vi "night.vi"() -> ()   [LabVIEW 2020]
uses:
  <vilib>/Analysis/baseanly.llb/Mean (DBL).vi
  <vilib>/Analysis/NI_AALBase.lvlib
panel:
  out "Error Out":errorcluster
  in  "milliseconds to wait":u32
  out "XY Graph":cluster{timestamp[], dbl[]}[](graph)
  in  "stop":bool
  out "Output":T1={"X"=[-0.192], "Y"=[-0.056], "Z"=[0.117], "Temperature"=0, "Timestamp"=525.141756172, "Digits"=3} {"Z" format="%.5f"; "Y" format="%.5f"; "X" format="%.5f"}
  in  "Select":T2={"X"=TRUE, "Y"=TRUE, "Z"=TRUE, "Temp"=FALSE, "Timstamp"=FALSE}
  out "File Error Out":errorcluster
  in  "COMMENT":string="BDC_z_reverse_D1_0A_D2_0A_SFDC_3A5"
  in  "base path":path=path "C:/LabVIEW/DATA/J-PARC_202403"
  in  "VISA resource":refnum<visa-resource-name>="USB0::0x1BFA::0x0498::0002759::INSTR"
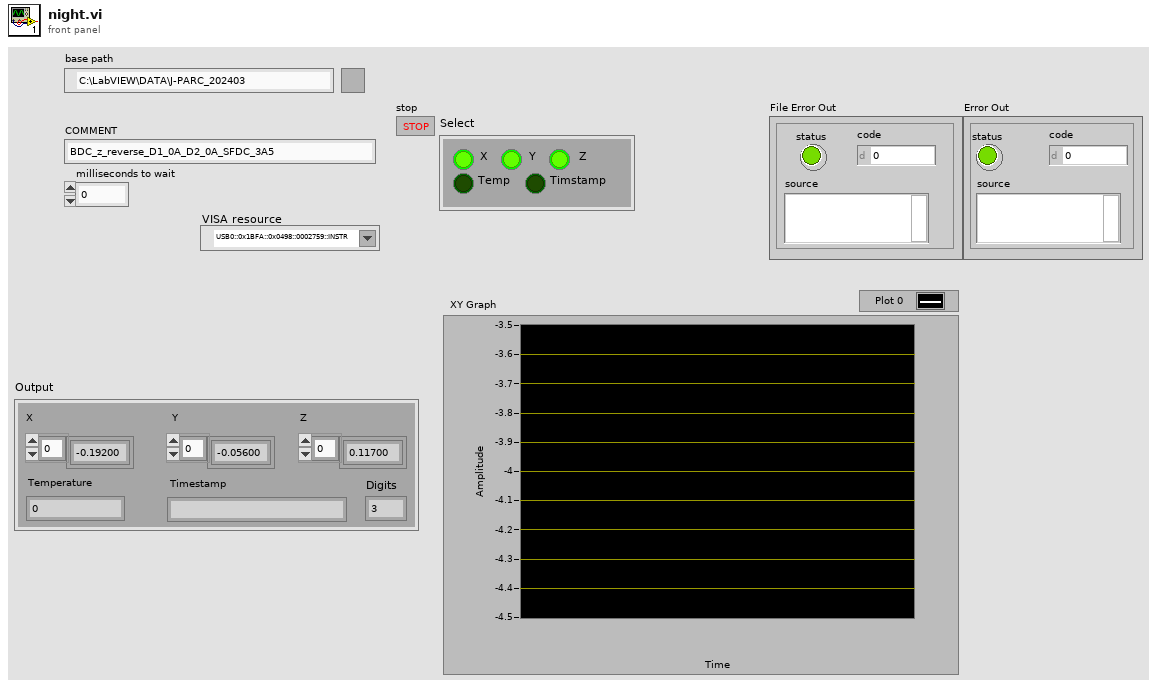
[diagram p1: front panel]
types:
  T1 = cluster{"X":dbl[], "Y":dbl[], "Z":dbl[], "Temperature":u16, "Timestamp":ext, "Digits":u8}
  T2 = cluster{"X":bool, "Y":bool, "Z":bool, "Temp":bool, "Timstamp":bool}
  T3 = enum16{"open", "replace", "create", "open or create", "replace or create", "replace or create with confirmation"}
  T4 = enum16{"Setup", "Setup query", "INITiate", "ABORt"}
  T5 = enum16{"Set units", "Units query", "Units all query"}
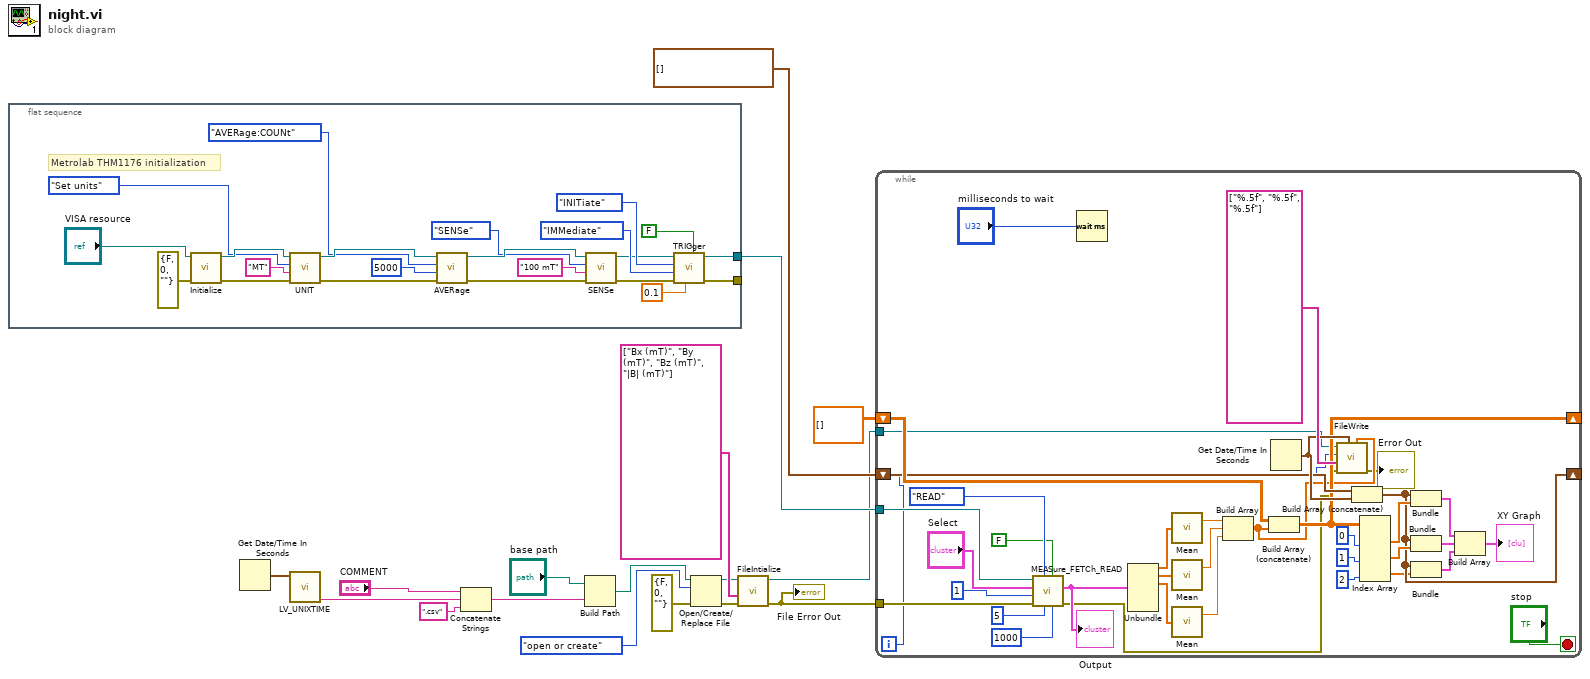
[diagram p0: block diagram]
diagram:
  n1 = flat-sequence {
    tunnel: [w25] -> w5
    tunnel: [w24] -> _
    frame #0 {
      # "Metrolab THM1176 initialization"
      n2 = call "Initialize.vi"("Error in (no error)"=errorcluster {"status"=FALSE, "code"=0, "source"=""}, "VISA resource"="VISA resource") -> ("Error out"=w36:errorcluster, "Dup VISA resource"=w37:refnum<visa-resource-name>)  [unwired: 3 in, 5 out]
      n3 = call "UNIT.vi"("Error in (no error)"=w36, "Units"="MT", "Function"=T5."Set units", "VISA resource"=w37) -> ("Error out"=w32:errorcluster, "Dup VISA resource"=w33:refnum<visa-resource-name>)  [unwired: 5 in, 1 out]
      n4 = call "AVERage.vi"("Error in (no error)"=w32, "Count"=u16 5000, "Function"=enum16{"AVERage:COUNt query", "AVERage:COUNt"}."AVERage:COUNt", "VISA resource"=w33) -> ("Error out"=w23:errorcluster, "Dup VISA resource"=w20:refnum<visa-resource-name>)  [unwired: 5 in, 1 out]
      n5 = call "SENSe.vi"("Error in (no error)"=w23, "Range"="100 mT", "Function"=enum16{"SENSe", "SENSe Query"}."SENSe", "VISA resource"=w20) -> ("Error out"=w22:errorcluster, "Dup VISA resource"=w21:refnum<visa-resource-name>)  [unwired: 4 in, 2 out]
      n6 = call "TRIGger.vi"("Continuous"=FALSE, "Period (s)"=0.1, "Error in (no error)"=w22, "Source"=enum16{"IMMediate", "TIMer", "BUS"}."IMMediate", "Function"=T4."INITiate", "VISA resource"=w21) -> ("Error out"=w24:errorcluster, "Dup VISA resource"=w25:refnum<visa-resource-name>)  [unwired: 3 in, 1 out]
    }
  }
  n7 = Get Date/Time In Seconds() -> (seconds since 1Jan1904=w15:timestamp)
  n8 = call "LV_UNIXTIME.vi"("current time"=w15) -> ("date/time string"=w12:string)  [unwired: 9 in, 1 out]
  n9 = Concatenate Strings("COMMENT", w12, ".csv" ("string")) -> (w10:string)
  n10 = Build Path(base path="base path", name or relative path=w10) -> (appended path=w14:path)
  n11 = Open/Create/Replace File(file path (use dialog)=w14, error in=errorcluster {"status"=FALSE, "code"=0, "source"=""} ("エラー入力"), operation (0:open)=T3."open or create") -> (refnum out=w7:refnum<file>, error out=w8:errorcluster)  [unwired: 3 in, 1 out]
  n12 = call "FileIntialize.vi"("Error In"=w8, "Labels"=string[] ["Bx (mT)", "By (mT)", "Bz (mT)", "|B| (mT)"], "refnum in"=w7) -> ("Error Out"=w4:errorcluster, "File Refnum"=w1:refnum<file>)  [unwired: 7 in]
  "File Error Out" <- w4
  n13 = while {
    tunnel: w5 -> [w67]
    tunnel: w4 -> [w66]
    shift-right: [w57] -> _
    shift-left: dbl[][] [] -> [w61]
    shift-right: [w49] -> _
    shift-left: timestamp[] [] -> [w59]
    tunnel: w1 -> [w43]
    i -> [w42]
    stop <- "stop" stop-if-true
    n14 = call "MEASure_FETCh_READ.vi"("Timeout (ms)"=u32 1000, "Sleep"=FALSE, "Digits"=u8 5, "Function"=enum16{"MEASure", "READ", "FETCh"}."READ", "Error in (no error)"=w66, "Size"=u16 1, "Select"="Select", "VISA resource"=w67) -> ("Error out"=w41:errorcluster, "Output"=w71:T1)  [unwired: 1 in, 1 out]
    "Output" <- w71
    n15 = Wait (ms)(milliseconds to wait="milliseconds to wait") -> ()  [unwired: 1 out]
    n16 = Unbundle(w71) -> ("X"=w70:dbl[], "Y"=w69:dbl[], "Z"=w68:dbl[])  [unwired: 3 out]
    n17 = call-poly <vilib>:"Mean.vi"("X"=w70) -> ("mean"=w64:dbl)  [unwired: 1 out]
    n18 = call-poly <vilib>:"Mean.vi"("X"=w69) -> ("mean"=w63:dbl)  [unwired: 1 out]
    n19 = call-poly <vilib>:"Mean.vi"("X"=w68) -> ("mean"=w62:dbl)  [unwired: 1 out]
    n20 = Build Array(w64, w63, w62) -> (w44:dbl[])
    n21 = Build Array (concatenate)(w61, w44) -> (w57:dbl[][])
    n22 = Get Date/Time In Seconds() -> (seconds since 1Jan1904=w60:timestamp)
    n23 = call "FileWrite.vi"("DataArray"=w44, "Time Stamp"=w60, "Error In"=w41, "FileFormat"=string[] ["%.5f", "%.5f", "%.5f"], "Index"=w42, "refnum in"=w43) -> ("Error Out"=→"Error Out":errorcluster)  [unwired: 4 in, 1 out]
    n24 = Build Array (concatenate)(w59, w60) -> (w49:timestamp[])
    n25 = Index Array(array=w57, index (col) #1=0 ("disabled index (col)"), index (col) #2=1 ("index (col)"), index (col) #3=2 ("index (col)")) -> (element #1=w55:dbl[], element #2=w50:dbl[], element #3=w48:dbl[])  [unwired: 3 in]
    n26 = Bundle(w49, w55) -> (w53:cluster{timestamp[], dbl[]})  [unwired: 1 in]
    n27 = Bundle(w49, w50) -> (w47:cluster{timestamp[], dbl[]})  [unwired: 1 in]
    n28 = Bundle(w49, w48) -> (w46:cluster{timestamp[], dbl[]})  [unwired: 1 in]
    n29 = Build Array(w53, w47, w46) -> (→"XY Graph":cluster{timestamp[], dbl[]}[])
  }
